vi "test_Add Array Format .vi"(8 "error in (no error)":errorcluster, 11 "TestCase in":refnum<class "Instrument Addon Scripting API Channels Unit Tests.lvclass">) -> (0 "error out":errorcluster, 3 "TestCase out":refnum<class "Instrument Addon Scripting API Channels Unit Tests.lvclass">)   [LabVIEW 2018, in "Instrument Addon Scripting API Channels Unit Tests.lvclass"]
uses:
  Instrument Addon Scripting API Channels Unit Tests.lvclass
  APIs/Scripting API/TypeDefs/Array Format Settings.ctl
  APIs/Scripting API/TypeDefs/Array Element.ctl
  Addon/Addon Shared/SubVIs/Constants.vi
  <vilib>/NI/NI VeriStand Advanced SysDef API/_SubVIs/SysDef.Search.GUID.vi
  <vilib>/NI/NI VeriStand Advanced SysDef API/_SubVIs/SysDef.Search.GUIDs.vi
  APIs/Scripting API/Channels/Create Data Channel - Array - Format.vi
  <vilib>/NI Veristand/Custom Device API/Get Item Property (String).vi
  <vilib>/addons/_JKI Toolkits/VI Tester/TestCase.llb/TestCase.lvclass
  Instrument Addon Scripting API Test Assets/Instrument Addon Scripting API Test Assets.lvclass
  <vilib>/NI/NI VeriStand Advanced SysDef API/SysDef API/Advanced System Definition.lvlib
  Addon/Addon Shared/Instrument Addon Shared.lvlib
  APIs/Scripting API/Instrument Addon Scripting API.lvlib
  <vilib>/NI Veristand/Custom Device API/Custom Device API.lvlib
  C:/Program Files (x86)/National Instruments/LabVIEW 2018/vi.lib/addons/_JKI Toolkits/VI Tester/TestCase.llb/TestCase.lvclass
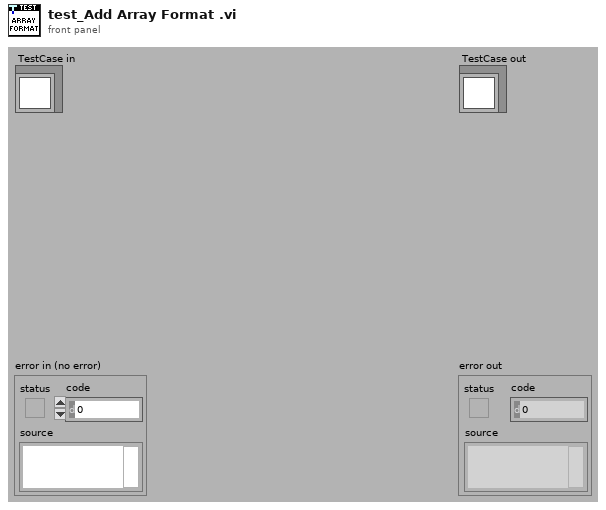
[diagram p1: front panel]
types:
  T1 = typedef "Instrument Addon Scripting API.lvlib/Array Format Settings.ctl" = cluster{"Elements":T2[], "Format String":string, "Delimiter":string}
  T2 = typedef "Instrument Addon Scripting API.lvlib/Array Element.ctl" = cluster{"Name":string, "Default Value":dbl, "Units":string}
  T3 = typedef "Custom Device API.lvlib/Custom Device Item Ref.ctl" = u64
  T4 = typedef "Advanced System Definition.lvlib/TreeItem.Info.ctl" = cluster{"Name":string, "Description":string, "GUID":string, "Is Channel":bool, "Channel":T5, "Is Waveform":bool, "Waveform":T7}
  T5 = typedef "Custom Device API.lvlib/Custom Device Channel.ctl" = cluster{"Type":T6, "Units":string, "Default Value":dbl, "Faultable":bool, "Scalable":bool}
  T6 = typedef "Custom Device API.lvlib/Custom Device Channel Type.ctl" = enum16{"Input", "Output"}
  T7 = typedef "Custom Device API.lvlib/Custom Device Waveform.ctl" = cluster{"Data Type":T8, "Units":string}
  T8 = typedef "Custom Device API.lvlib/Custom Device Waveform DataType.ctl" = enum16{"Double", "Complex Double"}
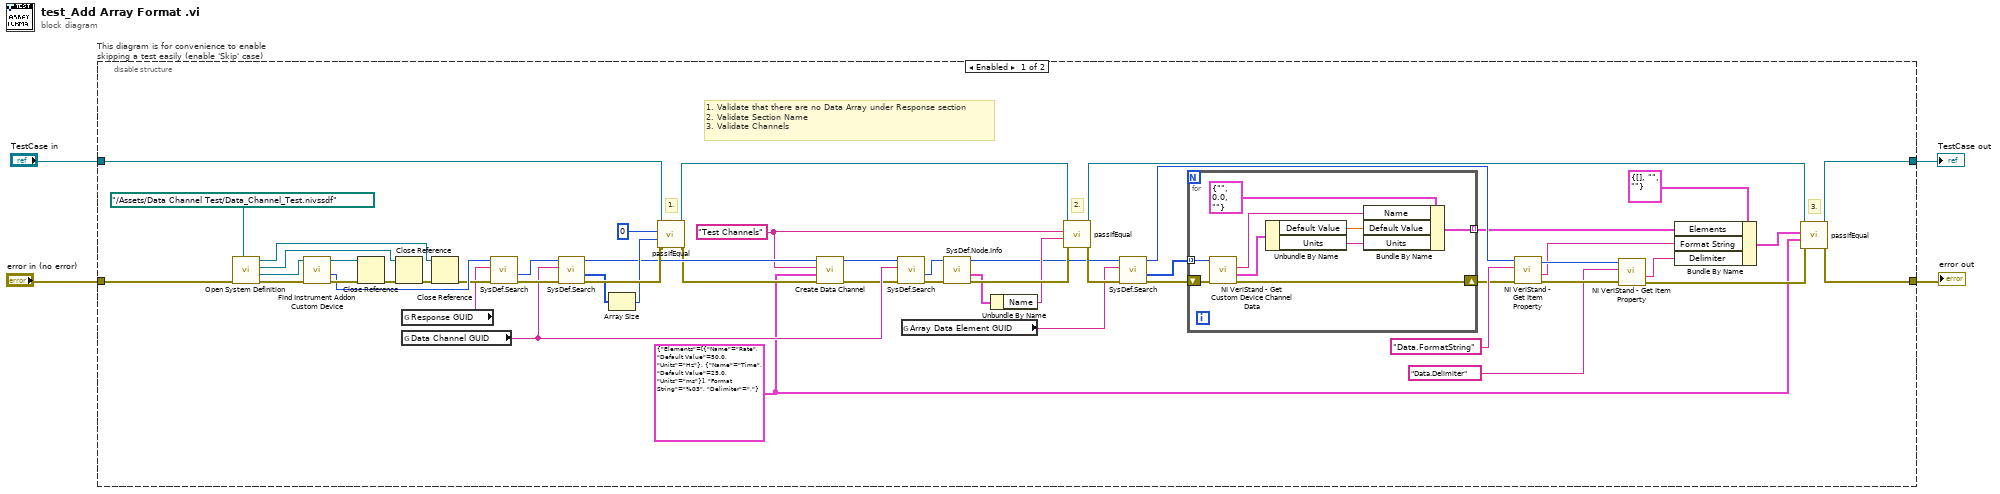
[diagram p0: block diagram]
diagram:
  n1 = disable-structure "This diagram is for convenience to enable skipping a test easily (enable 'Skip' case)" shown="Enabled" {
    disable-tunnel: "TestCase in" -> [w41 w70]
    disable-tunnel: [w19 w68] -> w1
    disable-tunnel: [w20 w69] -> w3
    disable-tunnel: "error in (no error)" -> [w48 w67]
    frame Enabled {
      w5 = T1 {"Elements"=[{"Name"="Rate", "Default Value"=50.0, "Units"="Hz"}, {"Name"="Time", "Default Value"=25.0, "Units"="ms"}], "Format String"="%03", "Delimiter"=","} ("Settings")
      w34 = "Test Channels" ("Name")
      # "3."
      # "2."
      # "1. Validate that there are no Data Array under Response section\n2. Validate Section Name\n3. Validate Channels"
      # "1."
      n2 = call "Open System Definition.vi"("error in (no error)"=w48, "System Definition File"=path "../Assets/Data Channel Test/Data_Channel_Test.nivssdf") -> ("error out"=w57:errorcluster, "Target Refnum"=w56:refnum<k24>, "Root Refnum"=w52:refnum<k24>, "System Definition Refnum"=w53:refnum<k24>)  [unwired: 6 in]
      n3 = call "Find Instrument Addon Custom Device.vi"("error in"=w57, "target in"=w56) -> ("error out"=w49:errorcluster, "NodeID"=w47:u64, "target out"=w50:refnum<k24>)  [unwired: 7 in]
      n4 = Close Reference(reference=w50, error in (no error)=w49) -> (error out=w51:errorcluster)
      n5 = Close Reference(reference=w52, error in (no error)=w51) -> (error out=w54:errorcluster)
      n6 = global read "Constants.vi" "Response GUID"() -> (w45:string)
      n7 = global read "Constants.vi" "Data Channel GUID"() -> (w42:string)
      n8 = Close Reference(reference=w53, error in (no error)=w54) -> (error out=w46:errorcluster)
      n9 = call-poly <vilib>:"SysDef.Search.vi"("error in (no error)"=w46, "GUID"=w45, "nodeID"=w47) -> ("error out"=w43:errorcluster, "Value out"=w44:u64)  [unwired: 5 in, 2 out]
      n10 = call-poly <vilib>:"SysDef.Search.vi"("error in (no error)"=w43, "GUID"=w42, "nodeID"=w44) -> ("error out"=w39:errorcluster, "Values Out"=w38:u64[], "nodeID out"=w35:u64)  [unwired: 5 in, 1 out]
      n11 = Array Size(array=w38) -> (size(s)=w37:i32)
      n12 = call-dynamic "passIfEqual.vi"("error in (no error)"=w39, "y"=w37, "x"=0 ("size(s)"), "TestCase in"=w41) -> ("error out"=w33:errorcluster, "TestCase out"=w40:refnum<class "Instrument Addon Scripting API Channels Unit Tests.lvclass">)  [unwired: 6 in]
      n13 = call-poly "Create Data Channel.vi"("Error In"=w33, "Settings"=w5, "Name"=w34, "Message Refnum In"=w35) -> ("Error Out"=w32:errorcluster, "Message Refnum Out"=w31:T3)  [unwired: 5 in, 1 out]
      n14 = call-poly <vilib>:"SysDef.Search.vi"("error in (no error)"=w32, "GUID"=w42, "nodeID"=w31) -> ("error out"=w30:errorcluster, "Value out"=w29:u64)  [unwired: 5 in, 2 out]
      n15 = global read "Constants.vi" "Array Data Element GUID"() -> (w22:string)
      n16 = call <vilib>:"SysDef.Node.Info.vi"("error in (no error)"=w30, "nodeID"=w29) -> ("error out"=w28:errorcluster, "Item Info"=w27:T4, "nodeID out"=w23:u64)  [unwired: 6 in, 1 out]
      n17 = Unbundle By Name(w27) -> ("Name"=w26:string)
      n18 = call-dynamic "passIfEqual.vi"("error in (no error)"=w28, "y"=w26, "x"=w34, "TestCase in"=w40) -> ("error out"=w25:errorcluster, "TestCase out"=w8:refnum<class "Instrument Addon Scripting API Channels Unit Tests.lvclass">)  [unwired: 6 in]
      n19 = call-poly <vilib>:"SysDef.Search.vi"("error in (no error)"=w25, "GUID"=w22, "nodeID"=w23) -> ("error out"=w24:errorcluster, "Values Out"=w21:u64[], "nodeID out"=w16:u64)  [unwired: 5 in, 1 out]
      n20 = for {
        shift-right: [w58] -> w17
        shift-left: w24 -> [w65]
        tunnel: w21 -> [w66] mode=indexing
        tunnel: [w59] -> w15 mode=indexing
        n21 = call <vilib>:"NI VeriStand - Get Custom Device Channel Data.vi"("error in (no error)"=w65, "Channel Ref in"=w66) -> ("error out"=w58:errorcluster, "Channel"=w62:T5, "Channel Name"=w63:string)  [unwired: 4 in, 3 out]
        n22 = Unbundle By Name(w62) -> ("Default Value"=w60:dbl, "Units"=w61:string)
        n23 = Bundle By Name(cluster=T2 {"Name"="", "Default Value"=0.0, "Units"=""} ("Array Element"), "Name"=w63, "Default Value"=w60, "Units"=w61) -> (w59:T2)
      }
      n24 = call-poly <vilib>:"NI VeriStand - Get Item Property.vi"("error in (no error)"=w17, "Property Name"="Data.FormatString", "Item Ref in"=w16) -> ("error out"=w14:errorcluster, "Value"=w6:string, "Item Ref out"=w13:T3)  [unwired: 5 in, 1 out]
      n25 = call-poly <vilib>:"NI VeriStand - Get Item Property.vi"("error in (no error)"=w14, "Property Name"="Data.Delimiter", "Item Ref in"=w13) -> ("error out"=w10:errorcluster, "Value"=w11:string)  [unwired: 5 in, 2 out]
      n26 = Bundle By Name(cluster=T1 {"Elements"=[], "Format String"="", "Delimiter"=""} ("Settings"), "Elements"=w15, "Format String"=w6, "Delimiter"=w11) -> (w9:T1)
      n27 = call-dynamic "passIfEqual.vi"("error in (no error)"=w10, "y"=w5, "x"=w9, "TestCase in"=w8) -> ("error out"=w20:errorcluster, "TestCase out"=w19:refnum<class "Instrument Addon Scripting API Channels Unit Tests.lvclass">)  [unwired: 6 in]
    }
    frame Disabled {
      # "skip test result while test is under development"
      n28 = call <vilib>:"skip.vi"("error in (no error)"=w67, "TestCase in"=w70) -> ("error out"=w69:errorcluster, "TestCase out"=w68:refnum<class "Instrument Addon Scripting API Channels Unit Tests.lvclass">)  [unwired: 8 in]
    }
  }
  "error out" <- w3
  "TestCase out" <- w1
